vi "Get Library Info.vi"(8 "error in (no error)":errorcluster {"code" format="Error %.0f"}, 11 "Library Documentation In":refnum<class "Library Documentation.lvclass">) -> (0 "error out":errorcluster {"code" format="Error %.0f"}, 2 "Library Info":T1, 3 "Library Documentation Out":refnum<class "Library Documentation.lvclass">)   [LabVIEW 2023, in "VIDoc Parsing.lvlib" / "Library Documentation.lvclass"]
uses:
  Library Documentation.lvclass
  TypeDefs/Base Library Info Cluster.ctl
  <vilib>/picture/picture.llb/imagedata.ctl
  Library Documentation.lvclass/Library Documentation.ctl
  VIDoc Parsing.lvlib
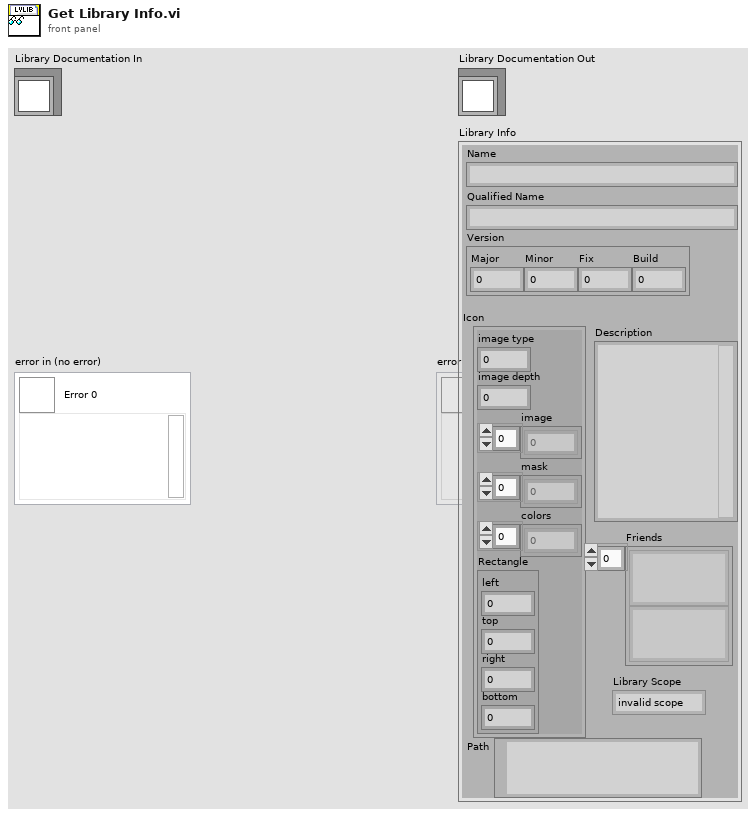
[diagram p1: front panel]
types:
  T1 = typedef "VIDoc Parsing.lvlib/Base Library Info Cluster.ctl" = cluster{"Name":string, "Icon":T2, "Version":cluster{"Major":u16, "Minor":u16, "Fix":u16, "Build":u16}, "Description":string, "Path":path, "Friends":string[], "Library Scope":enum32{"invalid scope", "public", "private", "protected", "community"}, "Qualified Name":string}
  T2 = typedef "imagedata.ctl" = cluster{"image type":i32, "image depth":i32, "image":u8[], "mask":u8[], "colors":u32[], "Rectangle":cluster{"left":i16, "top":i16, "right":i16, "bottom":i16}}
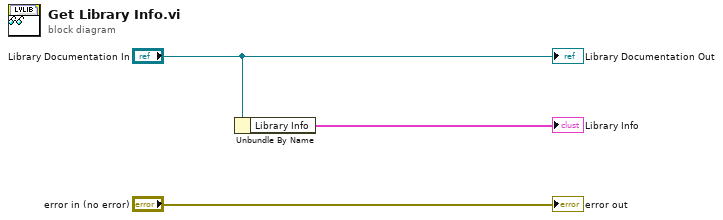
[diagram p0: block diagram]
diagram:
  n1 = Unbundle By Name("Library Documentation In") -> ("Library Info"=→"Library Info":T1)
  "error out" <- "error in (no error)"
  "Library Documentation Out" <- "Library Documentation In"
